vi "Stop.vi"(8 "error in (no error)":errorcluster, 11 "RP Instrument in":refnum<class "RP Instrument.lvclass">) -> (0 "error out":errorcluster, 3 "RP Instrument out":refnum<class "RP Instrument.lvclass">)   [LabVIEW 2015, in "RP Instrument.lvclass"]
uses:
  RP Instrument.lvclass
  RP Instrument.lvclass/RP Instrument.ctl
  RP Communicator/RP Communicator.lvclass
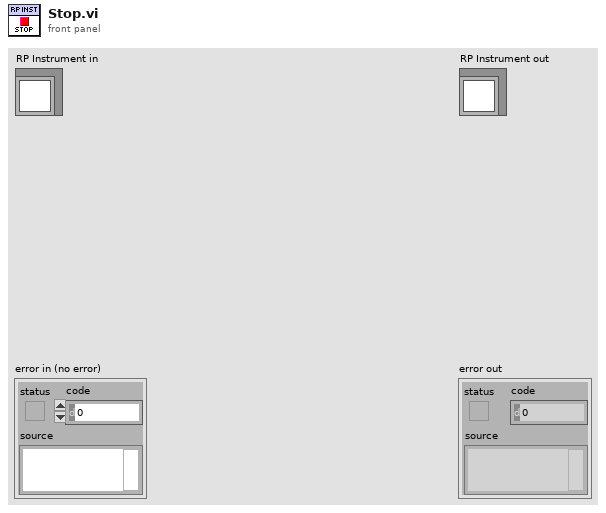
[diagram p1: front panel]
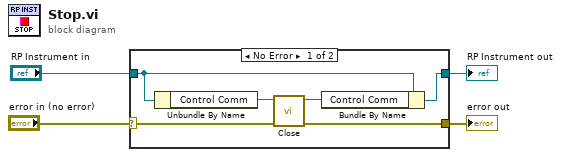
[diagram p0: block diagram]
diagram:
  n1 = case shown="No Error" "error in (no error)" {
    selector: "error in (no error)" -> [w6 w12]
    tunnel: [w5 w12] -> w3
    tunnel: [w8 w11] -> w1
    tunnel: "RP Instrument in" -> [w10 w11]
    frame No Error {
      n2 = Unbundle By Name(w10) -> ("Control Comm"=w9:refnum<class "RP Communicator.lvclass">)
      n3 = call-dynamic "Close.vi"("error in (no error)"=w6, "RP Communicator in"=w9) -> ("error out"=w5:errorcluster, "RP Communicator out"=w7:refnum<class "RP Communicator.lvclass">)  [unwired: 8 in]
      n4 = Bundle By Name(cluster=w10, "Control Comm"=w7) -> (w8:refnum<class "RP Instrument.lvclass">)
    }
    frame Error {
    }
  }
  "error out" <- w3
  "RP Instrument out" <- w1
